vi "FHT PtByPt.vi"(2 "initialize":bool, 3 "sample length":i32=100, 5 "x":dbl format="%0.2f") -> (0 "error":i32, 1 "Hartley{X}":dbl[](array[numeric]))   [LabVIEW 2020, in "NI_PtbyPt.lvlib"]
doc: "Computes the fast Hartley transform (FHT) of the set of input data points specified by <B>sample length</B>."
uses:
  <vilib>/ptbypt/NI_PtbyPt.lvlib
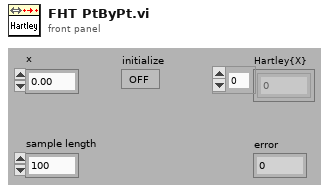
[diagram p1: front panel]
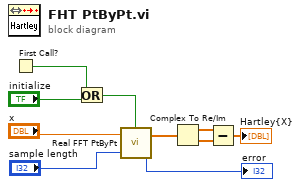
[diagram p0: block diagram]
diagram:
  n1 = First Call?() -> (First Call?: T/F=w1:bool)
  n2 = Or(x=w1, y="initialize") -> (x .or. y?=w2:bool)
  n3 = call <vilib>:"Real FFT PtByPt.vi"("initialize"=w2, "sample length"="sample length", "x"="x") -> ("error"=→"error":i32, "FFT{X}"=w3:cdb[])  [unwired: 1 in]
  n4 = Complex To Re/Im(x + iy=w3) -> (x=w10:dbl[], y=w9:dbl[])
  n5 = Subtract(x=w10, y=w9) -> (x-y=→"Hartley{X}":dbl[])
